vi "resultsColumns7HP.vi"(9 "7HP Probe Number":i32, 10 "Channel Values in":string[](array[string]), 11 "Channel Names in":string[](array[string])) -> (2 "Channel Values out":string[](array[string]), 3 "Channel Names out":string[](array[string]))   [LabVIEW 2022 SP3]
uses:
  Analysis/7 Hole Probe pressures to UVW/7HP_Global.vi
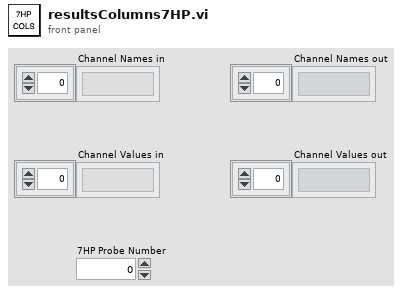
[diagram p1: front panel]
types:
  T1 = typedef "Correlation_cluster1.ctl" = cluster{"U inst":string, "uw":dbl, "u^2w":dbl, "uw^2":dbl, "uw/u'w'":dbl, "W inst":string, "uw^3":dbl, "u^3w":dbl, "u^2w^2":dbl, "Index U":i32, "Index W":i32, "Error info":string[], "Paired Sampling Rate (Hz)":dbl, "u^2 Paired":dbl, "w^2 Paired":dbl, "Time Window (ms)":dbl}
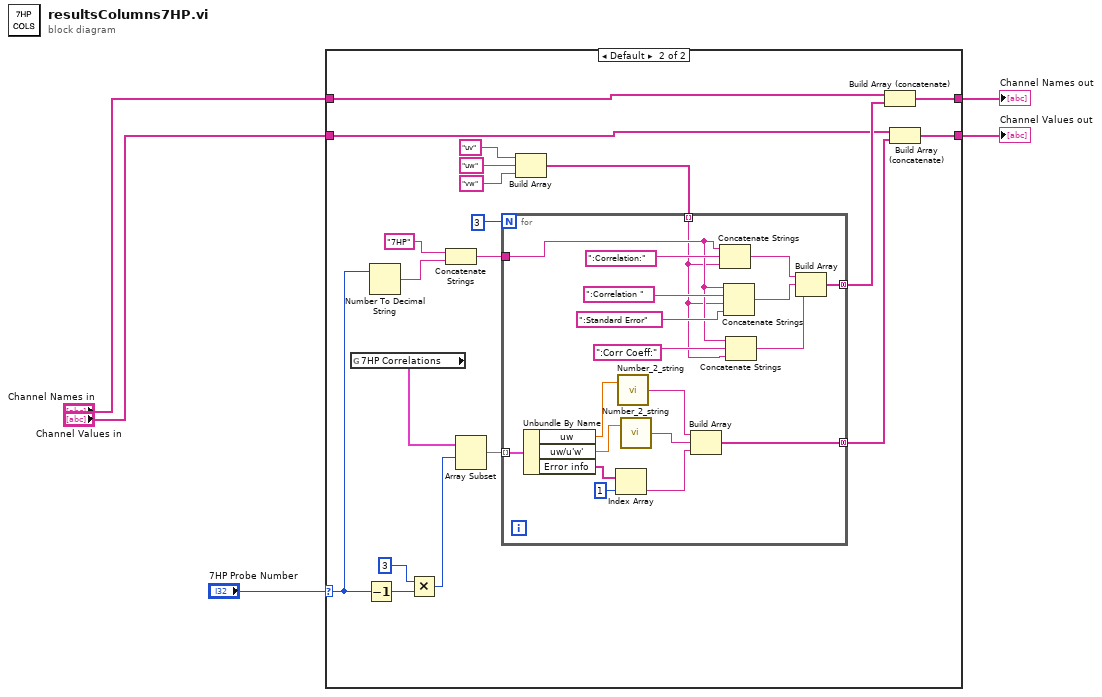
[diagram p0: block diagram]
diagram:
  n1 = case shown="Default" "7HP Probe Number" {
    selector: "7HP Probe Number" -> [_ w8]
    tunnel: "Channel Names in" -> [w7 w14]
    tunnel: "Channel Values in" -> [w6 w12]
    tunnel: [w7 w10] -> w5
    tunnel: [w6 w9] -> w4
    frame 0 {
    }
    frame Default {
      n2 = global read "7HP_Global.vi" "7HP Correlations"() -> (w24:T1[])
      n3 = Decrement(x=w8) -> (x-1=w27:i32)
      n4 = Number To Decimal String(number=w8) -> (decimal integer string=w20:string)  [unwired: 1 in]
      n5 = Multiply(x=3, y=w27) -> (x*y=w23:i32)
      n6 = Concatenate Strings("7HP" ("string"), w20) -> (w16:string)
      n7 = Array Subset(array=w24, index=w23) -> (w22:T1[])  [unwired: 1 in]
      n8 = Build Array("uv", "uw", "vw") -> (w15:string[])
      n9 = for {
        N: 3 -> [_]
        tunnel: w22 -> [w46] mode=indexing
        tunnel: w16 -> [w35]
        tunnel: w15 -> [w33] mode=indexing
        tunnel: [w29] -> w13 mode=concatenating
        tunnel: [w28] -> w11 mode=concatenating
        n10 = Unbundle By Name(w46) -> ("uw"=w43:dbl, "uw/u'w'"=w42:dbl, "Error info"=w45:string[])
        n11 = Index Array(array=w45, index=1) -> (element=w39:string)
        n12 = call "Number_2_string.vi"("number"=w43) -> ("String"=w41:string)  [unwired: 1 in]
        n13 = call "Number_2_string.vi"("number"=w42) -> ("String"=w40:string)  [unwired: 1 in]
        n14 = Build Array(w41, w40, w39) -> (w28:string[])
        n15 = Concatenate Strings(w35, ":Correlation:", w33) -> (w32:string)
        n16 = Concatenate Strings(w35, ":Correlation ", w33, ":Standard Error") -> (w31:string)
        n17 = Concatenate Strings(w35, ":Corr Coeff:", w33) -> (w30:string)
        n18 = Build Array(w32, w31, w30) -> (w29:string[])
      }
      n19 = Build Array (concatenate)(w14, w13) -> (w10:string[])
      n20 = Build Array (concatenate)(w12, w11) -> (w9:string[])
    }
  }
  "Channel Names out" <- w5
  "Channel Values out" <- w4
